vi "Get Database List of Names and Paths.vi"(8 "error in":errorcluster, 11 "Databases section Ref":T1 format="%.0x") -> (0 "error out":errorcluster, 1 "Paths":path[](array[path]), 2 "Names":string[](array[string]), 3 "Databases section Ref out":T1 format="%.0x")   [LabVIEW 2020, in "Ballard ARINC 429 Scripting.lvlib"]
uses:
  Ballard ARINC 429 Scripting.lvlib
  <vilib>/NI VeriStand/Custom Device API/Custom Device Item Ref.ctl
  <vilib>/NI VeriStand/Custom Device Tools/Custom Device Utility Library/Search Direction.ctl
  Constants.vi
  <vilib>/NI VeriStand/Custom Device Tools/Custom Device Utility Library/NI VeriStand - Search for Item by GUID.vi
  <vilib>/NI VeriStand/Custom Device API/Get Item Property (Path).vi
  <vilib>/NI VeriStand/Custom Device API/Custom Device API.lvlib
  <vilib>/NI VeriStand/Custom Device Tools/Custom Device Utility Library/Custom Device Utility Library.lvlib
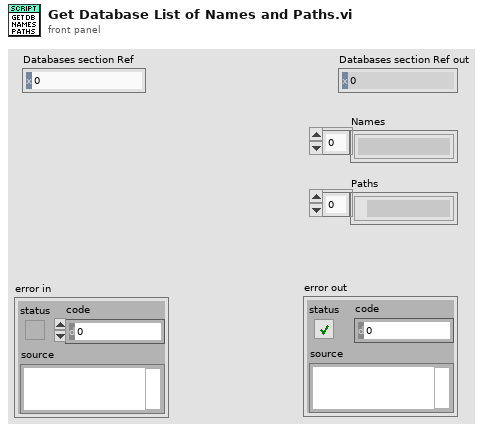
[diagram p1: front panel]
types:
  T1 = typedef "Custom Device API.lvlib/Custom Device Item Ref.ctl" = u64
  T2 = typedef "Custom Device Utility Library.lvlib/Search Direction.ctl" = enum16{"Down", "Up"}
  T3 = typedef "Custom Device API.lvlib/Custom Device Item Info.ctl" = cluster{"Name":string, "Is Channel":bool, "GUID":string, "Is Waveform":bool}
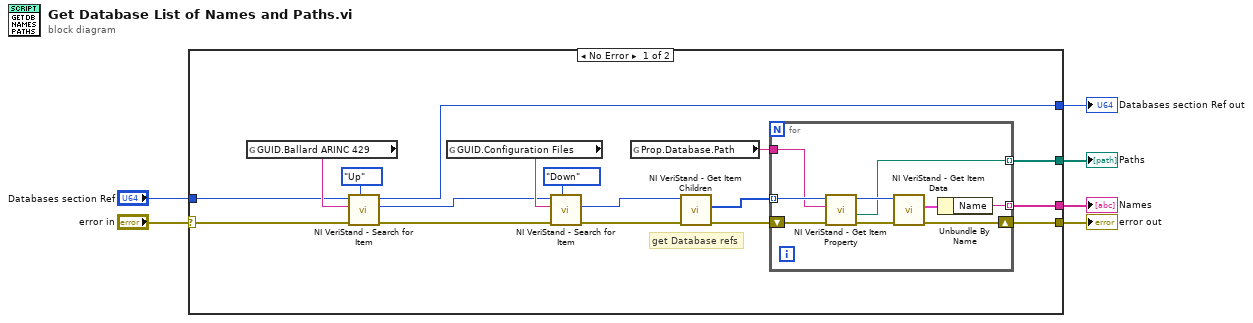
[diagram p0: block diagram]
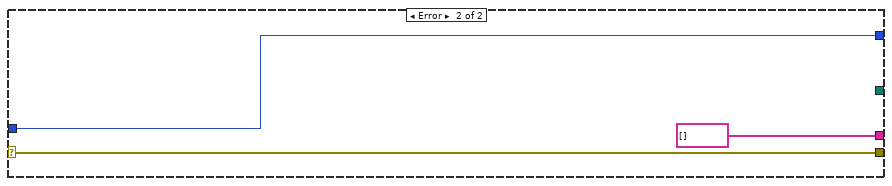
[diagram p2: hidden frame]
diagram:
  n1 = case shown="No Error" "error in" {
    selector: "error in" -> [w9 w35]
    tunnel: "Databases section Ref" -> [w19 w34]
    tunnel: [w18 w34] -> w5
    tunnel: [w11 string[] []] -> w4
    tunnel: [w10 w35] -> w3
    tunnel: [w7 _] -> w1
    frame No Error {
      # "get Database refs"
      n2 = global read "Constants.vi" "GUID.Ballard ARINC 429"() -> (w21:string)
      n3 = call-poly <vilib>:"NI VeriStand - Search for Item.vi"("Direction (Down)"=Search_Direction."Up", "error in"=w9, "Item GUID"=w21, "Section Ref in"=w19) -> ("error out"=w15:errorcluster, "Item Ref"=w16:T1, "Section Ref out"=w18:T1)  [unwired: 4 in, 1 out]
      n4 = global read "Constants.vi" "GUID.Configuration Files"() -> (w20:string)
      n5 = call-poly <vilib>:"NI VeriStand - Search for Item.vi"("Direction (Down)"=Search_Direction."Down", "error in"=w15, "Item GUID"=w20, "Section Ref in"=w16) -> ("error out"=w14:errorcluster, "Item Ref"=w17:T1)  [unwired: 4 in, 2 out]
      n6 = global read "Constants.vi" "Prop.Database.Path"() -> (w8:string)
      n7 = call <vilib>:"NI VeriStand - Get Item Children.vi"("error in (no error)"=w14, "Item Ref in"=w17) -> ("error out"=w12:errorcluster, "Child Refs"=w13:T1[])  [unwired: 6 in, 2 out]
      n8 = for {
        tunnel: w13 -> [w26] mode=indexing
        shift-right: [w31] -> w10
        shift-left: w12 -> [w29]
        tunnel: [w30] -> w11 mode=indexing
        tunnel: w8 -> [w25]
        tunnel: [w24] -> w7 mode=indexing
        n9 = call-poly <vilib>:"NI VeriStand - Get Item Property.vi"("error in (no error)"=w29, "Property Name"=w25, "Item Ref in"=w26) -> ("error out"=w28:errorcluster, "Value"=w24:path, "Item Ref out"=w27:T1)  [unwired: 5 in, 1 out]
        n10 = call <vilib>:"NI VeriStand - Get Item Data.vi"("error in (no error)"=w28, "Item Ref in"=w27) -> ("error out"=w31:errorcluster, "Item Info"=w32:T3)  [unwired: 6 in, 2 out]
        n11 = Unbundle By Name(w32) -> ("Name"=w30:string)
      }
    }
    frame Error {
    }
  }
  "Names" <- w4
  "error out" <- w3
  "Databases section Ref out" <- w5
  "Paths" <- w1
